vi "AO采样率检查与转化.vi"(8 "error in (no error)":errorcluster, 11 "AO FIFO Sample Rate":dbl=1000.0 min=1000.0 max=1600000.0) -> (0 "error out":errorcluster, 3 "Count (tick/s)":u32)   [LabVIEW 2019]
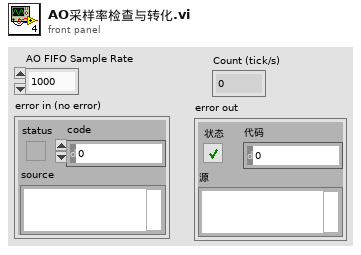
[diagram p1: front panel]
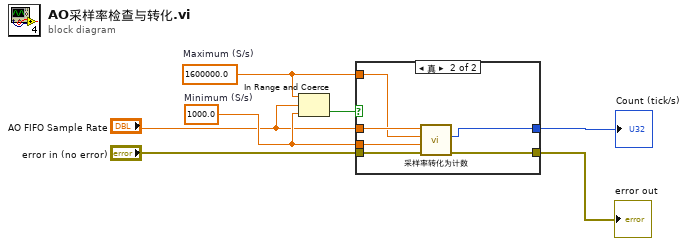
[diagram p0: block diagram]
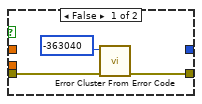
[diagram p2: hidden frame]
diagram:
  w5 = 1000.0  # Minimum (S/s)
  w7 = 1600000.0  # Maximum (S/s)
  n1 = In Range and Coerce(upper limit=w7, x="AO FIFO Sample Rate", lower limit=w5) -> (In Range?=w6:bool)  [unwired: 1 out]
  n2 = case shown="真" w6 {
    tunnel: [_ w12] -> w1
    tunnel: "error in (no error)" -> [w9 w13]
    tunnel: [w8 w11] -> w2
    tunnel: "AO FIFO Sample Rate" -> [_ w16]
    tunnel: w5 -> [_ w14]
    tunnel: w7 -> [_ w15]
    frame False {
      n3 = call <vilib>:"Error Cluster From Error Code.vi"("error in (no error)"=w9, "error code (0)"=-363040) -> ("error out"=w8:errorcluster)  [unwired: 7 in]
    }
    frame True {
      n4 = call "采样率转化为计数.vi"("Sample Rate (S/s)"=w16, "Maximum (S/s)"=w15, "Minimum (S/s)"=w14, "error in (no error)"=w13) -> ("Count (tick/s)"=w12:u32, "error out"=w11:errorcluster)  [unwired: 4 in, 1 out]
    }
  }
  "error out" <- w2
  "Count (tick/s)" <- w1
